vi "Write XY Plot ref.vi"(8 "error in (no error)":errorcluster, 10 "XY Plot ref":refnum<vi>, 11 "Instrument Actor in":refnum<class "Instrument Actor.lvclass">) -> (0 "error out":errorcluster, 3 "Instrument Actor out":refnum<class "Instrument Actor.lvclass">)   [LabVIEW 2024, in "Instrument Actor.lvclass"]
uses:
  Instrument Actor.lvclass
  Instrument Actor.lvclass/Instrument Actor.ctl
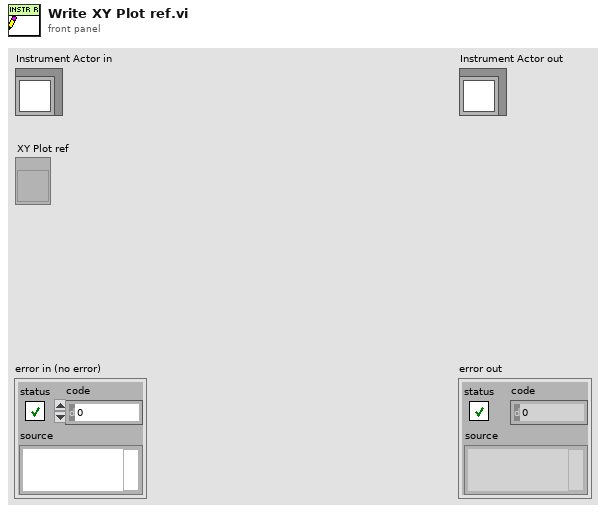
[diagram p1: front panel]
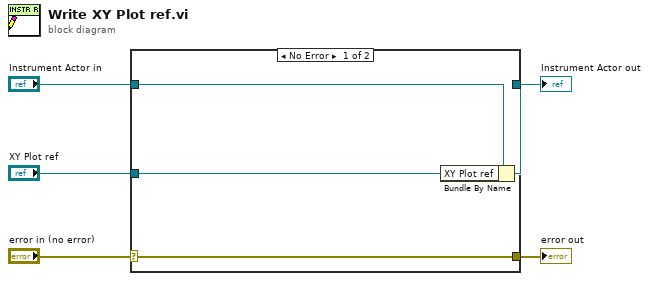
[diagram p0: block diagram]
diagram:
  n1 = case shown="No Error" "error in (no error)" {
    selector: "error in (no error)" -> [w9 w10]
    tunnel: [w9 w10] -> w4
    tunnel: [w7 w11] -> w2
    tunnel: "Instrument Actor in" -> [w8 w11]
    tunnel: "XY Plot ref" -> [w6 _]
    frame No Error {
      n2 = Bundle By Name(cluster=w8, "XY Plot ref"=w6) -> (w7:refnum<class "Instrument Actor.lvclass">)
    }
    frame Error {
    }
  }
  "error out" <- w4
  "Instrument Actor out" <- w2
